vi "IT8800-Initialize.vi"(8 "error in (no error)":errorcluster, 11 "ITech Setting In":T2={"VISA Resource Name"="", "Baud Rate"=19200, "Stop Bits"=20, "Wait For Read(ms)"=0, "Interface Type"=enum."VXI", "Limits"=[]} {"Stop Bits" items=["1.0"=10, "2.0"=20]; "Baud Rate" items=["2400"=2400, "4800"=4800, "9600"=9600, "19200"=19200]}) -> (0 "error out":errorcluster, 3 "IT8800 Setting In Out":T2={"VISA Resource Name"="", "Baud Rate"=19200, "Stop Bits"=20, "Wait For Read(ms)"=0, "Interface Type"=enum."VXI", "Limits"=[]} {"Stop Bits" items=["1.0"=10, "2.0"=20]; "Baud Rate" items=["2400"=2400, "4800"=4800, "9600"=9600, "19200"=19200]})   [LabVIEW 2018]
doc: "Establishes communication with the instrument and optionally performs an instrument identification query and/or an instrument reset. It also places the instrument in a default state needed for other instrument driver operations. Therefore, call this VI before calling other instrument driver VIs for this instrument. Generally, you need to call the Initialize VI only once at the beginning of an application."
uses:
  Data Def/IT8800-Setting.ctl
  Data Def/IT8800-Operation Mode.ctl
panel:
  in  "Range Type":T1
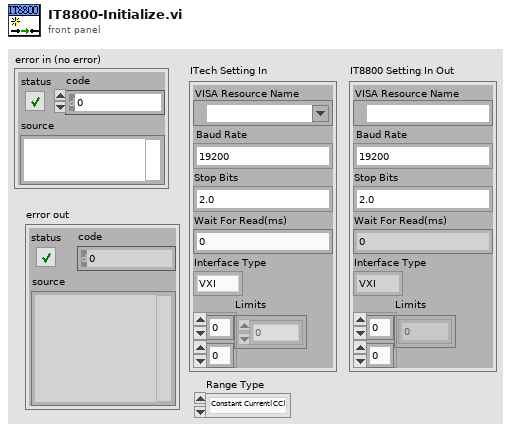
[diagram p1: front panel]
types:
  T1 = typedef "IT8800-Operation Mode.ctl" = enum16{"Constant Current(CC)", "Constant Voltage(CV)", "Constant Power(CP)", "Constant Resistance(CR)"}
  T2 = typedef "IT8800-Setting.ctl" = cluster{"VISA Resource Name":refnum<visa-resource-name>, "Baud Rate":u32, "Stop Bits":u16, "Wait For Read(ms)":u32, "Interface Type":enum16{"Unknow", "GPIB", "VXI", "GPIB-VXI", "Serial", "PXI", "TCPIP", "USB", "FireWire"}, "Limits":dbl[][]}
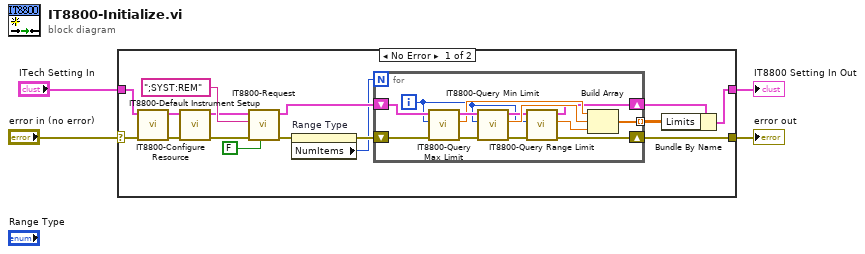
[diagram p0: block diagram]
diagram:
  n1 = case shown="No Error" "error in (no error)" {
    selector: "error in (no error)" -> [w13 w35]
    tunnel: [w11 w35] -> w4
    tunnel: [w8 w34] -> w3
    tunnel: "ITech Setting In" -> [w15 w34]
    frame No Error {
      n2 = call "IT8800-Configure Resource.vi"("error in (no error)"=w13, "ITech Setting In in"=w15) -> ("error out"=w17:errorcluster, "ITech Setting In out"=w14:T2)  [unwired: 8 in]
      n3 = call "IT8800-Default Instrument Setup.vi"("error in"=w17, "IT8800 Setting In In"=w14) -> ("error out"=w19:errorcluster, "IT8800 Setting In Out"=w18:T2)  [unwired: 8 in]
      n4 = call "IT8800-Request.vi"("Response?"=FALSE, "error in"=w19, "Command"=";SYST:REM" ("string"), "IT8800 Setting In In"=w18) -> ("error out"=w5:errorcluster, "IT8800 Setting In Out"=w12:T2)  [unwired: 5 in, 1 out]
      n5 = property on="Range Type" class="Enum (strict)"(error in=w5) -> (error out=w10:errorcluster, "NumItems"=w6:u32)  [unwired: 1 in, 1 out]
      n6 = for {
        N: w6 -> [_]
        shift-right: [w23] -> w9
        shift-left: w12 -> [w33]
        shift-right: [w22] -> w11
        shift-left: w10 -> [w32]
        tunnel: [w27] -> w7 mode=indexing
        i -> [w25]
        n7 = call "IT8800-Query Max Limit.vi"("error in"=w32, "Range Type"=w25, "IT8800 Setting In In"=w33) -> ("error out"=w30:errorcluster, "Range"=w29:dbl, "IT8800 Setting In Out"=w31:T2)  [unwired: 6 in]
        n8 = call "IT8800-Query Min Limit.vi"("error in"=w30, "Range Type"=w25, "IT8800 Setting In In"=w31) -> ("error out"=w24:errorcluster, "Range"=w28:dbl, "IT8800 Setting In Out"=w26:T2)  [unwired: 6 in]
        n9 = call "IT8800-Query Range Limit.vi"("error in"=w24, "Range Type"=w25, "IT8800 Setting In In"=w26) -> ("error out"=w22:errorcluster, "Range"=w21:dbl, "IT8800 Setting In Out"=w23:T2)  [unwired: 6 in]
        n10 = Build Array(w29, w28, w21) -> (w27:dbl[])
      }
      n11 = Bundle By Name(cluster=w9, "Limits"=w7) -> (w8:T2)
    }
    frame Error {
    }
  }
  "error out" <- w4
  "IT8800 Setting In Out" <- w3
